vi "ReadExpectedDependencies.vi"(8 "error in (no error)":errorcluster, 10 "Library Name":string, 11 "Build Specs Folder Path":path) -> (0 "error out":errorcluster, 1 "ExpectedDeps Path":path, 2 "Found?":bool, 3 "ExpectedDependencies":string[](array[string]))   [LabVIEW 2023, in "Reusables.lvlib"]
uses:
  Reusables.lvlib
  <userlib>/_OpenG.lib/file/file.llb/File Exists - Scalar__ogtk.vi
  <userlib>/_OpenG.lib/file/file.llb/openg_file.lvlib
  <vilib>/Utility/config.llb/NI_LVConfig.lvlib
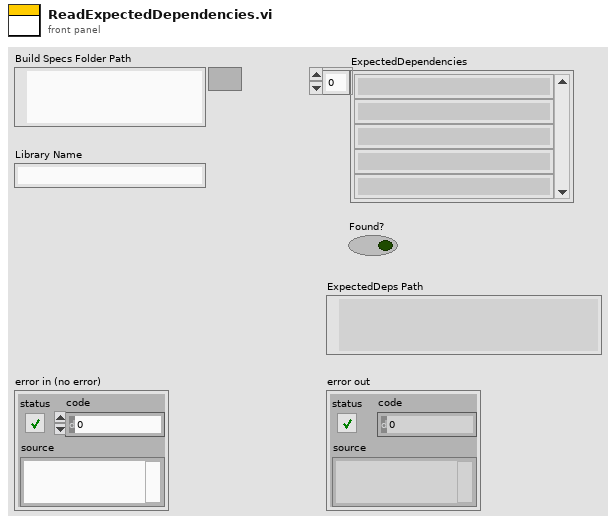
[diagram p1: front panel]
types:
  T1 = typedef "NI_LVConfig.lvlib/Config Data RefNum.ctl" = refnum<k1>
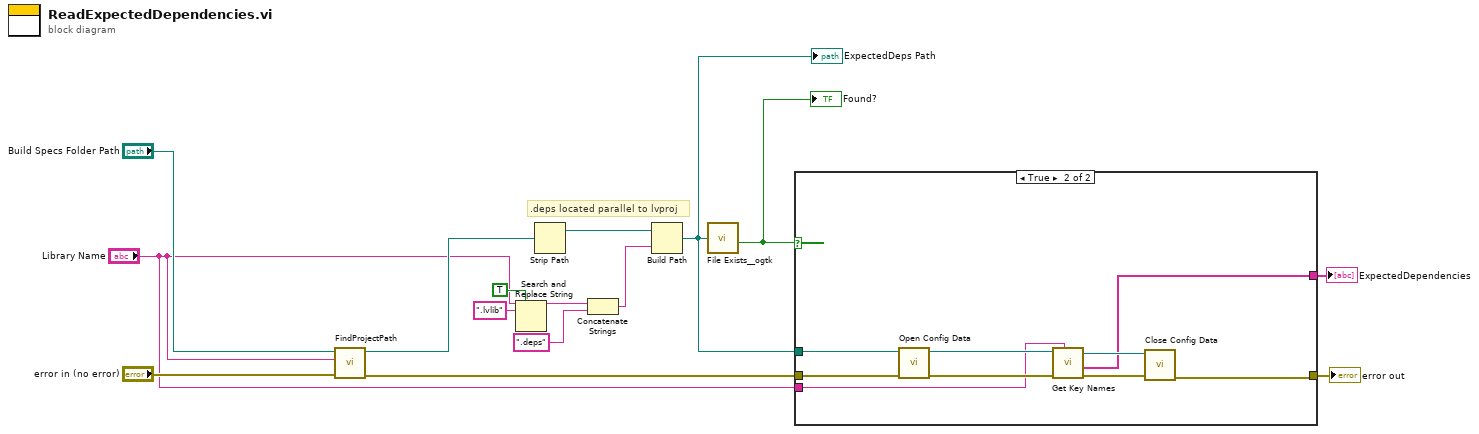
[diagram p0: block diagram]
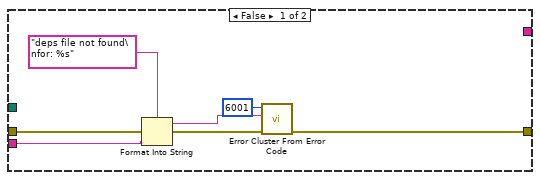
[diagram p2: hidden frame]
diagram:
  # ".deps located parallel to lvproj"
  n1 = call "FindProjectPath.vi"("error in (no error)"="error in (no error)", "Library Name"="Library Name", "Build Specs Folder Path"="Build Specs Folder Path") -> ("error out"=w6:errorcluster, "Project Path"=w13:path)  [unwired: 6 in, 1 out]
  n2 = Search and Replace String(replace all?=TRUE ("replace all? (F)"), input string="Library Name", search string=".lvlib") -> (result string=w9:string)  [unwired: 5 in, 3 out]
  n3 = Strip Path(path=w13) -> (stripped path=w12:path)  [unwired: 1 out]
  n4 = Concatenate Strings(w9, ".deps" ("string")) -> (w7:string)
  n5 = Build Path(base path=w12, name or relative path=w7) -> (appended path=w2:path)
  "ExpectedDeps Path" <- w2
  n6 = call-poly <userlib>:"File Exists__ogtk.vi"("file path"=w2) -> ("exists"=w1:bool)  [unwired: 6 in, 1 out]
  "Found?" <- w1
  n7 = case shown="True" w1 {
    tunnel: w6 -> [w21 w31]
    tunnel: "Library Name" -> [w19 w27]
    tunnel: [w16 w23] -> w4
    tunnel: w2 -> [_ w30]
    tunnel: [_ w24] -> w3
    frame False {
      n8 = Format Into String(format string="deps file not found\nfor: %s" ("error message (\"\")"), error in=w21, w19) -> (resulting string=w18:string, error out=w17:errorcluster)  [unwired: 1 in]
      n9 = call <vilib>:"Error Cluster From Error Code.vi"("error in (no error)"=w17, "error message (\"\")"=w18, "error code (0)"=6001) -> ("error out"=w16:errorcluster)  [unwired: 6 in]
    }
    frame True {
      n10 = call <vilib>:"Open Config Data.vi"("error in (no error)"=w31, "configuration file path"=w30) -> ("error out"=w29:errorcluster, "refnum"=w28:T1)  [unwired: 7 in, 1 out]
      n11 = call <vilib>:"Get Key Names.vi"("section"=w27, "error in (no error)"=w29, "refnum"=w28) -> ("error out"=w26:errorcluster, "key names"=w24:string[], "refnum out"=w25:T1)  [unwired: 5 in, 1 out]
      n12 = call <vilib>:"Close Config Data.vi"("error in (no error)"=w26, "refnum"=w25) -> ("error out"=w23:errorcluster)  [unwired: 8 in, 1 out]
    }
  }
  "error out" <- w4
  "ExpectedDependencies" <- w3
